vi "Shock&Dyanamics Laboratory - DROPBEAR_June2022_Rev3.vi"() -> ()   [LabVIEW 2019] (continued)
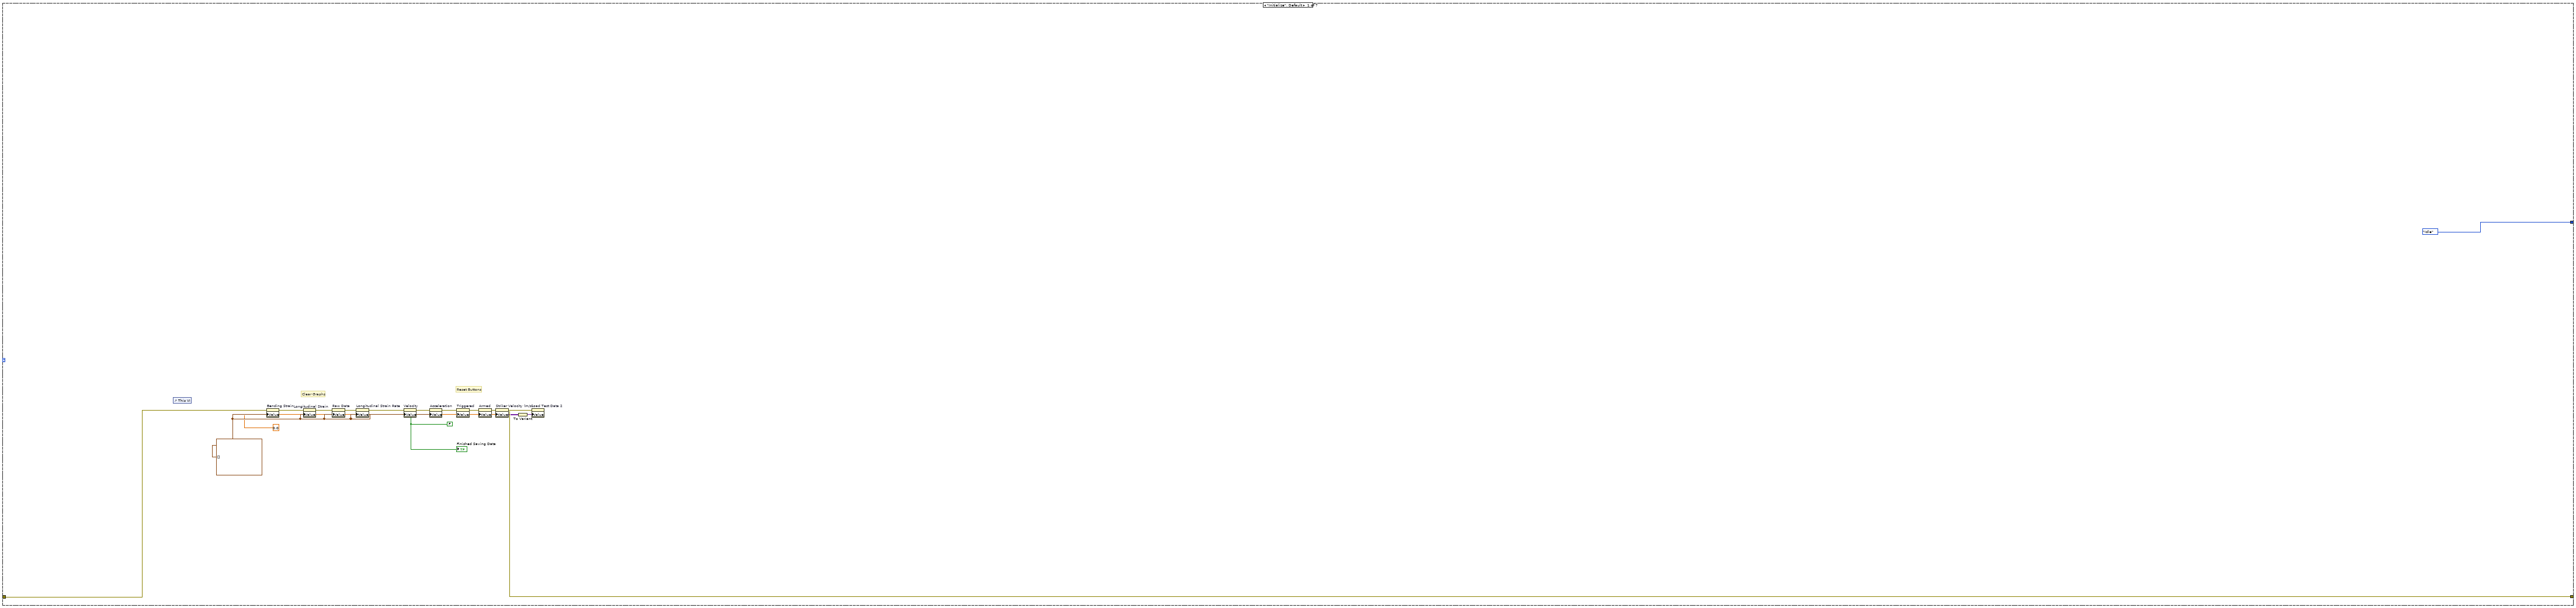
[diagram p2: hidden frame]
                # "== Need to change save file to accuratly save the sperated and strain-rate Data =="
                n2032 = Two Button Dialog(message="Use the folder/file names already given?", 1:"No" ("F button name (\"Cancel\")"), 2:"Yes" ("T button name (\"OK\")")) -> (T button?=w2561:bool)
                n2033 = case shown="True" w2561 {
                  tunnel: [w2582 "Folder Name to Save Raw Data"] -> w2560
                  tunnel: [w2581 "File Name to Save Raw Data"] -> w2559
                  tunnel: w2558 -> [w2579 w2583]
                  tunnel: [w2578 w2583] -> w2557
                  frame False {
                    n2034 = call "32CHDAQ - New FileFolder Names.vi"("Enable"=TRUE, "error in (no error)"=w2579) -> ("File Name (don't forget .txt)"=w2581:string, "Folder Name"=w2582:string, "error out"=w2578:errorcluster)  [unwired: 14 in, 1 out]
                  }
                  frame True {
                  }
                }
                n2035 = flat-sequence {
                  tunnel: w2557 -> [w2586]
                  tunnel: w2559 -> [w2587]
                  tunnel: w2560 -> [w2588]
                  tunnel: [w2588] -> w2572
                  tunnel: [w2587] -> w2571
                  tunnel: [w2586] -> w2570
                  tunnel: [w2592] -> w2556
                  tunnel: [w2594] -> w2554
                  tunnel: [w2593] -> w2552
                  tunnel: w2572 -> [w2594]
                  tunnel: w2571 -> [w2593]
                  tunnel: w2570 -> [w2591]
                  tunnel: w2573 -> [w2590]
                  tunnel: [w2590] -> w2550
                  tunnel: w2556 -> [w2609]
                  tunnel: [w2608] -> w2555
                  tunnel: w2554 -> [w2606]
                  tunnel: [w2606] -> w2553
                  tunnel: w2552 -> [w2607]
                  tunnel: [w2607] -> w2551
                  tunnel: w2550 -> [w2605]
                  tunnel: [w2605] -> w2549
                  tunnel: "Incident Name for First Pulse\n(Must Match Exactly" -> [w2604]
                  tunnel: w2555 -> [w2628]
                  tunnel: w2553 -> [w2623]
                  tunnel: w2551 -> [w2629]
                  tunnel: [w2623] -> w2569
                  tunnel: [w2629] -> w2568
                  tunnel: [w2627] -> w2567
                  tunnel: w2549 -> [w2626]
                  tunnel: [w2626] -> w2566
                  tunnel: "Incident Name for First Pulse\n(Must Match Exactly" -> [w2624]
                  tunnel: w2569 -> [w2659]
                  tunnel: w2568 -> [w2658]
                  tunnel: [w2659] -> w2565
                  tunnel: [w2658] -> w2564
                  tunnel: [w2656] -> w2563
                  tunnel: w2567 -> [w2657]
                  tunnel: w2566 -> [w2655]
                  tunnel: [w2655] -> w2562
                  tunnel: w2565 -> [w2678]
                  tunnel: w2564 -> [w2677]
                  tunnel: w2563 -> [w2676]
                  tunnel: [w2675] -> w2574
                  tunnel: w2562 -> [w2674]
                  frame #0 {
                  }
                  frame #1 {
                    w2589 = TRUE
                    # "Saves Raw Data"
                    n2036 = case shown="True" w2589 {
                      tunnel: w2594 -> [_ w2603]
                      tunnel: w2593 -> [_ w2602]
                      tunnel: [w2595 w2601] -> w2592
                      tunnel: w2591 -> [w2595 w2599]
                      tunnel: w2590 -> [_ w2597]
                      frame False {
                      }
                      frame True {
                        n2037 = property on="Raw Data" class="WFGraph (strict)"() -> ("Value"=w2596:waveform(dbl)[])  [unwired: 2 in, 2 out]
                        n2038 = property on="Save Info" class="Clust (strict)"() -> ("Value"=w2598:T5)  [unwired: 2 in, 2 out]
                        n2039 = Concatenate Strings(w2603, w2602) -> (w2600:string)
                        n2040 = call "32CHDAQ - Save Data File 0 Raw.vi"("Save Info"=w2598, "error in"=w2599, "waveforms"=w2596, "output cluster 3"=w2597, "File name"=w2600) -> ("error out"=w2601:errorcluster)  [unwired: 6 in]
                      }
                    }
                    "?" <- w2589
                  }
                  frame #2 {
                    # "Saves First Pulse of Raw Data"
                    n2041 = case shown="True" "First Pulse" {
                      tunnel: w2609 -> [w2611 w2621]
                      tunnel: [w2611 w2620] -> w2608
                      tunnel: w2607 -> [_ w2617]
                      tunnel: w2606 -> [_ w2616]
                      tunnel: w2605 -> [_ w2615]
                      tunnel: w2604 -> [_ w2612]
                      frame False {
                      }
                      frame True {
                        # "Save First Pulse Only subVI"
                        n2042 = property on="Raw Data" class="WFGraph (strict)"() -> ("Value"=w2613:waveform(dbl)[])  [unwired: 2 in, 2 out]
                        n2043 = Concatenate Strings(w2616, "First_Pulse_" ("string"), w2617) -> (w2618:string)
                        n2044 = property on="Save Info" class="Clust (strict)"() -> ("Value"=w2614:T5)  [unwired: 2 in, 2 out]
                        n2045 = call "32CHDAQ - Save Data File - FirstPulse.vi"("Incident Name for First Pulse\n(Must Match Exactly"=w2612, "Save Info"=w2614, "error in"=w2621, "waveforms"=w2613, "output cluster 3"=w2615, "File name"=w2618) -> ("error out"=w2620:errorcluster)  [unwired: 5 in]
                      }
                    }
                  }
                  frame #3 {
                    n2046 = property on="First Pulse" class="Bool (strict)"() -> ("Value"=w2622:bool)  [unwired: 2 in, 2 out]
                    n2047 = case shown="True" "?" {
                      tunnel: w2623 -> [_ w2635]
                      tunnel: w2629 -> [_ w2636]
                      tunnel: w2628 -> [w2630 w2640]
                      tunnel: [w2630 w2639] -> w2627
                      tunnel: w2626 -> [_ w2632]
                      tunnel: w2624 -> [_ w2637]
                      tunnel: w2622 -> [_ w2631]
                      frame False {
                      }
                      frame True {
                        (unwired) "Scaled Data" ("Comment")
                        n2048 = property on="Scaled Data" class="Arr (strict)"() -> ("Value"=w2634:waveform(dbl)[])  [unwired: 2 in, 2 out]
                        n2049 = Concatenate Strings(w2635, "True_" ("string"), w2636) -> (w2641:string)
                        n2050 = property on="Save Info" class="Clust (strict)"() -> ("Value"=w2633:T5)  [unwired: 2 in, 2 out]
                        n2051 = call "32CHDAQ - Save Data File.vi"("Save Info"=w2633, "error in"=w2640, "waveforms"=w2634, "output cluster 3"=w2632, "File name"=w2641) -> ("error out"=w2638:errorcluster)  [unwired: 6 in]
                        n2052 = case shown="True" w2631 {
                          tunnel: w2638 -> [w2643 w2653]
                          tunnel: [w2643 w2652] -> w2639
                          tunnel: w2636 -> [_ w2649]
                          tunnel: w2635 -> [_ w2648]
                          tunnel: w2632 -> [_ w2647]
                          tunnel: w2637 -> [_ w2646]
                          tunnel: w2634 -> [_ w2645]
                          tunnel: w2633 -> [_ w2644]
                          frame False {
                          }
                          frame True {
                            # "Save First Pulse Only subVI"
                            n2053 = Concatenate Strings(w2648, "First_Pulse_Scaled_" ("string"), w2649) -> (w2650:string)
                            n2054 = call "32CHDAQ - Save Data File - FirstPulse.vi"("Incident Name for First Pulse\n(Must Match Exactly"=w2646, "Save Info"=w2644, "error in"=w2653, "waveforms"=w2645, "output cluster 3"=w2647, "File name"=w2650) -> ("error out"=w2652:errorcluster)  [unwired: 5 in]
                          }
                        }
                      }
                    }
                  }
                  frame #4 {
                    # "Saves Separated Data - Turned Off Right Now"
                    n2055 = case shown="True" "Separated" {
                      tunnel: w2659 -> [_ w2671]
                      tunnel: w2658 -> [_ w2670]
                      tunnel: w2657 -> [w2660 w2666]
                      tunnel: [w2660 w2665] -> w2656
                      tunnel: w2655 -> [_ w2661]
                      frame False {
                      }
                      frame True {
                        (unwired) "Seperated Data" ("Comment")
                        n2056 = property on="Bending Strain" class="WFGraph (strict)"() -> ("Value"=w2668:waveform(dbl)[])  [unwired: 2 in, 2 out]
                        n2057 = Concatenate Strings(w2671, "Sep_" ("string"), w2670) -> (w2663:string)
                        n2058 = property on="Longitudinal Strain" class="WFGraph (strict)"() -> ("Value"=w2669:waveform(dbl)[])  [unwired: 2 in, 2 out]
                        n2059 = Insert Into Array(array=waveform(dbl)[] [], new element #1=w2668, new element #2=w2669) -> (w2664:waveform(dbl)[])  [unwired: 1 in]
                        n2060 = property on="Save Info" class="Clust (strict)"() -> ("Value"=w2662:T5)  [unwired: 2 in, 2 out]
                        n2061 = call "32CHDAQ - Save Data File - Seperated.vi"("Save Info"=w2662, "error in"=w2666, "waveforms"=w2664, "output cluster 3"=w2661, "File name"=w2663) -> ("error out"=w2665:errorcluster)  [unwired: 6 in]
                      }
                    }
                  }
                  frame #5 {
                    # "Save Strain-Rate Data - Turned Off Right Now"
                    n2062 = case shown="True" "?" {
                      tunnel: w2678 -> [_ w2688]
                      tunnel: w2677 -> [_ w2687]
                      tunnel: w2676 -> [w2679 w2684]
                      tunnel: [w2679 w2683] -> w2675
                      tunnel: w2674 -> [_ w2681]
                      frame False {
                      }
                      frame True {
                        (unwired) "Strain Rate Data" ("Comment")
                        n2063 = Concatenate Strings(w2688, "Rate_" ("string"), w2687) -> (w2686:string)
                        n2064 = property on="Rate Data" class="Arr (strict)"() -> ("Value"=w2680:waveform(dbl)[])  [unwired: 2 in, 2 out]
                        n2065 = property on="Save Info" class="Clust (strict)"() -> ("Value"=w2685:T5)  [unwired: 2 in, 2 out]
                        n2066 = case shown="False" FALSE {
                          tunnel: w2686 -> [_ w2696]
                          tunnel: w2685 -> [_ w2695]
                          tunnel: w2680 -> [_ w2691]
                          tunnel: w2684 -> [w2690 w2694]
                          tunnel: [w2690 w2693] -> w2683
                          tunnel: w2681 -> [_ w2692]
                          frame False {
                          }
                          frame True {
                            n2067 = call "32CHDAQ - Save Data File - Rate.vi"("Save Info"=w2695, "error in"=w2694, "waveforms"=w2691, "output cluster 3"=w2692, "File name"=w2696) -> ("error out"=w2693:errorcluster)  [unwired: 6 in]
                          }
                        }
                      }
                    }
                  }
                }
              }
            }
            n2068 = property on="Finished Saving Data" class="Bool (strict)"(error in=w2543, "Value"=TRUE ("Finished Saving Data")) -> (error out=w2541:errorcluster)  [unwired: 1 in, 1 out]
            n2069 = property on="Triggered" class="Bool (strict)"(error in=w2541, "Value"=FALSE ("Triggered")) -> (error out=w2539:errorcluster)  [unwired: 1 in, 1 out]
            n2070 = flat-sequence {
              tunnel: w2539 -> [w2697]
              tunnel: [w2697] -> w2538
              frame #0 {
                n2071 = Wait (ms)(milliseconds to wait=u32 1000) -> ()  [unwired: 1 out]
              }
            }
          }
          frame "Load Data" {
            n2072 = Two Button Dialog(message="Have you loaded the associated Channel Data file?\n(if not, do so before loading the Test Data File)     ", 1:"No" ("F button name (\"Cancel\")"), 2:"Yes" ("T button name (\"OK\")")) -> (T button?=w2703:bool)
            n2073 = case shown="True" w2703 {
              tunnel: [32CHDAQ_-_Cases."Idle" ("Program State") 32CHDAQ_-_Cases."Process Data" ("Program State")] -> w2702
              frame False {
                n2074 = To Variant(anything=FALSE) -> (Variant=w2707:variant)
                n2075 = property on="Load Test Data 2" class="Bool"("Value"=w2707) -> ()  [unwired: 2 in, 2 out]
              }
              frame True {
                w2723 = T58 1 items=["no dialog", "OK message", "continue or stop message", "OK message + warnings", "continue/stop + warnings"] ("type of dialog (OK msg:1)")
                # "Prompt User to Load Test Data File"
                n2076 = property on="output cluster" class="Clust (strict)"() -> (error out=w2714:errorcluster, "Value"=w2715:T2)  [unwired: 2 in, 1 out]
                n2077 = property on="Folder Name to Save Raw Data" class="Str"() -> ("Value"=w2732:string)  [unwired: 2 in, 2 out]
                n2078 = Unbundle(w2715) -> (w2720:T59, w2719:T60)  [unwired: 10 out]
                n2079 = Cluster To Array(cluster=w2720) -> (array=w2716:bool[])
                n2080 = Cluster To Array(cluster=w2719) -> (array=w2718:string[])
                n2081 = String To Path(string=w2732) -> (path=w2733:path)
                n2082 = File Dialog(4:"TXT File" ("pattern label"), 6:"*.txt" ("pattern"), 7:"Load Channel Data File" ("prompt"), 9:"*.txt" ("default name"), 11:w2733) -> (3:w2709:path)  [unwired: 2 in, 3 out]
                n2083 = call-poly <vilib>:"Read Delimited Spreadsheet.vi"("file path (dialog if empty)"=w2709) -> ("all rows"=w2708:dbl[][])  [unwired: 9 in, 5 out]
                n2084 = Transpose 2D Array(2D array=w2708) -> (transposed array=w2712:dbl[][])
                n2085 = Delete From Array(array=w2712, length=9, index (col)=0 ("index")) -> (array with subset deleted=w2711:dbl[][])  [unwired: 1 in, 1 out]
                n2086 = for {
                  tunnel: w2718 -> [w2741] mode=indexing
                  shift-right: [w2740] -> w2727
                  shift-left: string[] [] -> [w2739]
                  tunnel: w2716 -> [w2738] mode=indexing
                  n2087 = case shown="True" w2738 {
                    tunnel: w2741 -> [_ w2743]
                    tunnel: [w2742 w2745] -> w2740
                    tunnel: w2739 -> [w2742 w2744]
                    frame False {
                    }
                    frame True {
                      n2088 = Build Array (concatenate)(w2744, w2743) -> (w2745:string[])
                    }
                  }
                }
                n2089 = property on="Sample Rate (Sa/sec)" class="DigNum (strict)"(error in=w2714) -> (error out=w2726:errorcluster, "Value"=w2731:dbl)  [unwired: 1 in, 1 out]
                n2090 = for {
                  N -> [w2752]
                  tunnel: w2711 -> [w2755] mode=indexing
                  tunnel: w2731 -> [w2753]
                  tunnel: [w2750] -> w2730 mode=indexing
                  tunnel: [w2752] -> w2729
                  tunnel: w2727 -> [w2748] mode=indexing
                  shift-right: [w2746] -> w2725
                  shift-left: w2726 -> [w2747]
                  n2091 = Reciprocal(x=w2753) -> (1/x=w2754:dbl)
                  n2092 = Bundle By Name("dt"=w2754, "Y"=w2755) -> (w2751:waveform(dbl))  [unwired: 1 in]
                  n2093 = Set Waveform Attribute(4:w2747, 5:w2748, 6:"NI_ChannelName" ("name"), 7:w2751) -> (0:w2746:errorcluster, 3:w2750:waveform(dbl))  [unwired: 1 out]
                }
                n2094 = property on="Raw Data" class="WFGraph (strict)"(error in=w2725, "Value"=w2730) -> (error out=w2724:errorcluster)  [unwired: 1 in, 1 out]
                n2095 = Decrement(x=w2729) -> (x-1=w2728:i32)
                n2096 = property on="Number of Channels" class="DigNum (strict)"(error in=w2724, "Value"=w2728) -> (error out=w2722:errorcluster)  [unwired: 1 in, 1 out]
                n2097 = call <vilib>:"Simple Error Handler.vi"("type of dialog (OK msg:1)"=w2723, "error in (no error)"=w2722) -> ()  [unwired: 3 in, 5 out]
              }
            }
          }
          frame "End" {
            w2757 = FALSE ("Finished Saving Data")
            w2759 = waveform(dbl)[] [] ("array")
            # "Reset Buttons"
            # "Clear  Graphs"
            # "This is just a placeholder"
            # "Tie Up any Loose ends before ending Program"
            n2098 = property on="Raw Data" class="WFGraph (strict)"(error in=w2766, "Value"=w2759) -> (error out=w2765:errorcluster)  [unwired: 1 in, 1 out]
            n2099 = property on="Longitudinal Strain" class="WFGraph (strict)"(error in=w2765, "Value"=w2759) -> (error out=w2764:errorcluster)  [unwired: 1 in, 1 out]
            n2100 = property on="Bending Strain" class="WFGraph (strict)"(error in=w2764, "Value"=w2759) -> (error out=w2763:errorcluster)  [unwired: 1 in, 1 out]
            n2101 = property on="Longitudinal Strain Rate" class="WFGraph (strict)"(error in=w2763, "Value"=w2759) -> (error out=w2762:errorcluster)  [unwired: 1 in, 1 out]
            n2102 = property on="Velocity" class="WFGraph (strict)"(error in=w2762, "Value"=w2759) -> (error out=w2761:errorcluster)  [unwired: 1 in, 1 out]
            n2103 = property on="Acceleration" class="WFGraph (strict)"(error in=w2761, "Value"=w2759) -> (error out=w2760:errorcluster)  [unwired: 1 in, 1 out]
            n2104 = property on="Finished Saving Data" class="Bool (strict)"(error in=w2760, "Value"=w2757) -> (error out=w2767:errorcluster)  [unwired: 1 in, 1 out]
            n2105 = call <vilib>:"Simple Error Handler.vi"("error in (no error)"=w2767) -> ("error out"=w2758:errorcluster)  [unwired: 4 in, 4 out]
            "Triggered" <- w2757
            "Armed" <- w2757
          }
        }
      }
      frame #1 {
        # "Add \nProperty\nNode\nHere"
        # "Gather Channel Information"
        n2106 = Bundle("Sens Fac 0"="Sens Fac 0", "Sens Fac 1"="Sens Fac 1", "Sens Fac 2"="Sens Fac 2", "Sens Fac 3"="Sens Fac 3", "Sens Fac 4"="Sens Fac 4", "Sens Fac 5"="Sens Fac 5", "Sens Fac 6"="Sens Fac 6", "Sens Fac 7"="Sens Fac 7", "Sens Fac 8"="Sens Fac 8", "Sens Fac 9"="Sens Fac 9", "Sens Fac 10"="Sens Fac 10", "Sens Fac 11"="Sens Fac 11", "Sens Fac 12"="Sens Fac 12", "Sens Fac 13"="Sens Fac 13", "Sens Fac 14"="Sens Fac 14", "Sens Fac 15"="Sens Fac 15", "Sens Fac 16"="Sens Fac 16", "Sens Fac 17"="Sens Fac 17", "Sens Fac 18"="Sens Fac 18", "Sens Fac 19"="Sens Fac 19", "Sens Fac 20"="Sens Fac 20", "Sens Fac 21"="Sens Fac 21", "Sens Fac 22"="Sens Fac 22", "Sens Fac 23"="Sens Fac 23", "Sens Fac 24"="Sens Fac 24", "Sens Fac 25"="Sens Fac 25", "Sens Fac 26"="Sens Fac 26", "Sens Fac 27"="Sens Fac 27", "Sens Fac 28"="Sens Fac 28", "Sens Fac 29"="Sens Fac 29", "Sens Fac 30"="Sens Fac 30", "Sens Fac 31"="Sens Fac 31") -> (w2984:T51)  [unwired: 1 in]
        n2107 = Bundle(TRUE, "Enable Ch 1"="Enable Ch 1", "Enable Ch 2"="Enable Ch 2", "Enable Ch 3"="Enable Ch 3", "Enable Ch 4"="Enable Ch 4", "Enable Ch 5"="Enable Ch 5", "Enable Ch 6"="Enable Ch 6", "Enable Ch 7"="Enable Ch 7", "Enable Ch 8"="Enable Ch 8", "Enable Ch 9"="Enable Ch 9", "Enable Ch 10"="Enable Ch 10", "Enable Ch 11"="Enable Ch 11", "Enable Ch 12"="Enable Ch 12", "Enable Ch 13"="Enable Ch 13", "Enable Ch 14"="Enable Ch 14", "Enable Ch 15"="Enable Ch 15", "Enable Ch 16"="Enable Ch 16", "Enable Ch 17"="Enable Ch 17", "Enable Ch 18"="Enable Ch 18", "Enable Ch 19"="Enable Ch 19", "Enable Ch 20"="Enable Ch 20", "Enable Ch 21"="Enable Ch 21", "Enable Ch 22"="Enable Ch 22", "Enable Ch 23"="Enable Ch 23", "Enable Ch 24"="Enable Ch 24", "Enable Ch 25"="Enable Ch 25", "Enable Ch 26"="Enable Ch 26", "Enable Ch 27"="Enable Ch 27", "Enable Ch 28"="Enable Ch 28", "Enable Ch 29"="Enable Ch 29", "Enable Ch 30"="Enable Ch 30", "Enable Ch 31"="Enable Ch 31") -> (w2989:T59)  [unwired: 1 in]
        "ON/OFF" <- w2989
        n2108 = Bundle("SG Pair Ch 0"="SG Pair Ch 0", "SG Pair Ch 1"="SG Pair Ch 1", "SG Pair Ch 2"="SG Pair Ch 2", "SG Pair Ch 3"="SG Pair Ch 3", "SG Pair Ch 4"="SG Pair Ch 4", "SG Pair Ch 5"="SG Pair Ch 5", "SG Pair Ch 6"="SG Pair Ch 6", "SG Pair Ch 7"="SG Pair Ch 7", "SG Pair Ch 8"="SG Pair Ch 8", "SG Pair Ch 9"="SG Pair Ch 9", "SG Pair Ch 10"="SG Pair Ch 10", "SG Pair Ch 11"="SG Pair Ch 11", "SG Pair Ch 12"="SG Pair Ch 12", "SG Pair Ch 13"="SG Pair Ch 13", "SG Pair Ch 14"="SG Pair Ch 14", "SG Pair Ch 15"="SG Pair Ch 15", "SG Pair Ch 16"="SG Pair Ch 16", "SG Pair Ch 17"="SG Pair Ch 17", "SG Pair Ch 18"="SG Pair Ch 18", "SG Pair Ch 19"="SG Pair Ch 19", "SG Pair Ch 20"="SG Pair Ch 20", "SG Pair Ch 21"="SG Pair Ch 21", "SG Pair Ch 22"="SG Pair Ch 22", "SG Pair Ch 23"="SG Pair Ch 23", "SG Pair Ch 24"="SG Pair Ch 24", "SG Pair Ch 25"="SG Pair Ch 25", "SG Pair Ch 26"="SG Pair Ch 26", "SG Pair Ch 27"="SG Pair Ch 27", "SG Pair Ch 28"="SG Pair Ch 28", "SG Pair Ch 29"="SG Pair Ch 29", "SG Pair Ch 30"="SG Pair Ch 30", "SG Pair Ch 31"="SG Pair Ch 31") -> (w2981:T53)  [unwired: 1 in]
        n2109 = Bundle("Voltage Max Ch 0"="Voltage Max Ch 0", "Voltage Max Ch 1"="Voltage Max Ch 1", "Voltage Max Ch 2"="Voltage Max Ch 2", "Voltage Max Ch 3"="Voltage Max Ch 3", "Voltage Max Ch 4"="Voltage Max Ch 4", "Voltage Max Ch 5"="Voltage Max Ch 5", "Voltage Max  Ch 6"="Voltage Max  Ch 6", "Voltage Max Ch 7"="Voltage Max Ch 7", "Voltage Max Ch 8"="Voltage Max Ch 8", "Voltage Max Ch 9"="Voltage Max Ch 9", "Voltage Max Ch 10"="Voltage Max Ch 10", "Voltage Max Ch 11"="Voltage Max Ch 11", "Voltage Max Ch 12"="Voltage Max Ch 12", "Voltage Max Ch 13"="Voltage Max Ch 13", "Voltage Max Ch 14"="Voltage Max Ch 14", "Voltage Max Ch 15"="Voltage Max Ch 15", "Voltage Max Ch 16"="Voltage Max Ch 16", "Voltage Max Ch 17"="Voltage Max Ch 17", "Voltage Max Ch 18"="Voltage Max Ch 18", "Voltage Max Ch 19"="Voltage Max Ch 19", "Voltage Max Ch 20"="Voltage Max Ch 20", "Voltage Max Ch 21"="Voltage Max Ch 21", "Voltage Max Ch 22"="Voltage Max Ch 22", "Voltage Max Ch 23"="Voltage Max Ch 23", "Voltage Max Ch 24"="Voltage Max Ch 24", "Voltage Max Ch 25"="Voltage Max Ch 25", "Voltage Max Ch 26"="Voltage Max Ch 26", "Voltage Max Ch 27"="Voltage Max Ch 27", "Voltage Max Ch 28"="Voltage Max Ch 28", "Voltage Max Ch 29"="Voltage Max Ch 29", "Voltage Max Ch 30"="Voltage Max Ch 30", "Voltage Max Ch 31"="Voltage Max Ch 31") -> (w2986:T61)  [unwired: 1 in]
        n2110 = Bundle("SG Pair 0"="SG Pair 0", "SG Pair 1"="SG Pair 1", "SG Pair 2"="SG Pair 2", "SG Pair 3"="SG Pair 3", "SG Pair 4"="SG Pair 4", "SG Pair 5"="SG Pair 5", "SG Pair 6"="SG Pair 6", "SG Pair 7"="SG Pair 7", "SG Pair 8"="SG Pair 8", "SG Pair 9"="SG Pair 9", "SG Pair 10"="SG Pair 10", "SG Pair 11"="SG Pair 11", "SG Pair 12"="SG Pair 12", "SG Pair 13"="SG Pair 13", "SG Pair 14"="SG Pair 14", "SG Pair 15"="SG Pair 15", "SG Pair 16"="SG Pair 16", "SG Pair 17"="SG Pair 17", "SG Pair 18"="SG Pair 18", "SG Pair 19"="SG Pair 19", "SG Pair 20"="SG Pair 20", "SG Pair 21"="SG Pair 21", "SG Pair 22"="SG Pair 22", "SG Pair 23"="SG Pair 23", "SG Pair 24"="SG Pair 24", "SG Pair 25"="SG Pair 25", "SG Pair 26"="SG Pair 26", "SG Pair 27"="SG Pair 27", "SG Pair 28"="SG Pair 28", "SG Pair 29"="SG Pair 29", "SG Pair 30"="SG Pair 30", "SG Pair 31"="SG Pair 31") -> (w2982:T52)  [unwired: 1 in]
        n2111 = Bundle("Name (Laser Gate)"="Name (Laser Gate)", "Name Ch 1"="Name Ch 1", "Name Ch 2"="Name Ch 2", "Name Ch 3"="Name Ch 3", "Name Ch 4"="Name Ch 4", "Name Ch 5"="Name Ch 5", "Name Ch 6"="Name Ch 6", "Name Ch 7"="Name Ch 7", "Name Ch 8"="Name Ch 8", "Name Ch 9"="Name Ch 9", "Name Ch 10"="Name Ch 10", "Name Ch 11"="Name Ch 11", "Name Ch 12"="Name Ch 12", "Name Ch 13"="Name Ch 13", "Name Ch 14"="Name Ch 14", "Name Ch 15"="Name Ch 15", "Name Ch 16"="Name Ch 16", "Name Ch 17"="Name Ch 17", "Name Ch 18"="Name Ch 18", "Name Ch 19"="Name Ch 19", "Name Ch 20"="Name Ch 20", "Name Ch 21"="Name Ch 21", "Name Ch 22"="Name Ch 22", "Name Ch 23"="Name Ch 23", "Name Ch 24"="Name Ch 24", "Name Ch 25"="Name Ch 25", "Name Ch 26"="Name Ch 26", "Name Ch 27"="Name Ch 27", "Name Ch 28"="Name Ch 28", "Name Ch 29"="Name Ch 29", "Name Ch 30"="Name Ch 30", "Name Ch 31"="Name Ch 31") -> (w2990:T60)  [unwired: 1 in]
        n2112 = Bundle("Voltage Min Ch 0"="Voltage Min Ch 0", "Voltage Min Ch 1"="Voltage Min Ch 1", "Voltage Min Ch 2"="Voltage Min Ch 2", "Voltage Min Ch 3"="Voltage Min Ch 3", "Voltage Min Ch 4"="Voltage Min Ch 4", "Voltage Min Ch 5"="Voltage Min Ch 5", "Voltage Min Ch 6"="Voltage Min Ch 6", "Voltage Min Ch 7"="Voltage Min Ch 7", "Voltage Min Ch 8"="Voltage Min Ch 8", "Voltage Min Ch 9"="Voltage Min Ch 9", "Voltage Min Ch 10"="Voltage Min Ch 10", "Voltage Min Ch 11"="Voltage Min Ch 11", "Voltage Min Ch 12"="Voltage Min Ch 12", "Voltage Min Ch 13"="Voltage Min Ch 13", "Voltage Min Ch 14"="Voltage Min Ch 14", "Voltage Min Ch 15"="Voltage Min Ch 15", "Voltage Min Ch 16"="Voltage Min Ch 16", "Voltage Min Ch 17"="Voltage Min Ch 17", "Voltage Min Ch 18"="Voltage Min Ch 18", "Voltage Min Ch 19"="Voltage Min Ch 19", "Voltage Min Ch 20"="Voltage Min Ch 20", "Voltage Min Ch 21"="Voltage Min Ch 21", "Voltage Min Ch 22"="Voltage Min Ch 22", "Voltage Min Ch 23"="Voltage Min Ch 23", "Voltage Min Ch 24"="Voltage Min Ch 24", "Voltage Min Ch 25"="Voltage Min Ch 25", "Voltage Min Ch 26"="Voltage Min Ch 26", "Voltage Min Ch 27"="Voltage Min Ch 27", "Voltage Min Ch 28"="Voltage Min Ch 28", "Voltage Min Ch 29"="Voltage Min Ch 29", "Voltage Min Ch 30"="Voltage Min Ch 30", "Voltage Min Ch 31"="Voltage Min Ch 31") -> (w2987:T62)  [unwired: 1 in]
        n2113 = Bundle("Signal Type 0"="Signal Type 0", "Signal Type 1"="Signal Type 1", "Signal Type 2"="Signal Type 2", "Signal Type 3"="Signal Type 3", "Signal Type 4"="Signal Type 4", "Signal Type 5"="Signal Type 5", "Signal Type 6"="Signal Type 6", "Signal Type 7"="Signal Type 7", "Signal Type 8"="Signal Type 8", "Signal Type 9"="Signal Type 9", "Signal Type 10"="Signal Type 10", "Signal Type 11"="Signal Type 11", "Signal Type 12"="Signal Type 12", "Signal Type 13"="Signal Type 13", "Signal Type 14"="Signal Type 14", "Signal Type 15"="Signal Type 15", "Signal Type 16"="Signal Type 16", "Signal Type 17"="Signal Type 17", "Signal Type 18"="Signal Type 18", "Signal Type 19"="Signal Type 19", "Signal Type 20"="Signal Type 20", "Signal Type 21"="Signal Type 21", "Signal Type 22"="Signal Type 22", "Signal Type 23"="Signal Type 23", "Signal Type 24"="Signal Type 24", "Signal Type 25"="Signal Type 25", "Signal Type 26"="Signal Type 26", "Signal Type 27"="Signal Type 27", "Signal Type 28"="Signal Type 28", "Signal Type 29"="Signal Type 29", "Signal Type 30"="Signal Type 30", "Signal Type 31"="Signal Type 31") -> (w2983:T4)  [unwired: 1 in]
        "Signal Type" <- w2983
        n2114 = call "16CHDAQ - PF Info Num2Str.vi"("PF Channel"="PF Card 0", "PF Card"="PF Channel 0", "PF Chassis"="PF Chassis 0") -> ("PF Info"=w3152:string)
        n2115 = call "16CHDAQ - PF Info Num2Str.vi"("PF Channel"="PF Card 1", "PF Card"="PF Channel 1", "PF Chassis"="PF Chassis 1") -> ("PF Info"=w3156:string)
        n2116 = call "16CHDAQ - PF Info Num2Str.vi"("PF Channel"="PF Channel 2", "PF Card"="PF Card 2", "PF Chassis"="PF Chassis 2") -> ("PF Info"=w3162:string)
        n2117 = call "16CHDAQ - PF Info Num2Str.vi"("PF Channel"="PF Channel 3", "PF Card"="PF Card 3", "PF Chassis"="PF Chassis 3") -> ("PF Info"=w3166:string)
        n2118 = call "16CHDAQ - PF Info Num2Str.vi"("PF Channel"="PF Channel 4", "PF Card"="PF Card 4", "PF Chassis"="PF Chassis 4") -> ("PF Info"=w3170:string)
        n2119 = call "16CHDAQ - PF Info Num2Str.vi"("PF Channel"="PF Channel 5", "PF Card"="PF Card 5", "PF Chassis"="PF Chassis 5") -> ("PF Info"=w3174:string)
        n2120 = call "16CHDAQ - PF Info Num2Str.vi"("PF Channel"="PF Channel 6", "PF Card"="PF Card 6", "PF Chassis"="PF Chassis 6") -> ("PF Info"=w3178:string)
        n2121 = call "16CHDAQ - PF Info Num2Str.vi"("PF Channel"="PF Channel 7", "PF Card"="PF Card 7", "PF Chassis"="PF Chassis 7") -> ("PF Info"=w3182:string)
        n2122 = call "16CHDAQ - PF Info Num2Str.vi"("PF Channel"="PF Channel 8", "PF Card"="PF Card 8", "PF Chassis"="PF Chassis 8") -> ("PF Info"=w3186:string)
        n2123 = call "16CHDAQ - PF Info Num2Str.vi"("PF Channel"="PF Channel 9", "PF Card"="PF Card 9", "PF Chassis"="PF Chassis 9") -> ("PF Info"=w3215:string)
        n2124 = call "16CHDAQ - PF Info Num2Str.vi"("PF Channel"="PF Channel 10", "PF Card"="PF Card 10", "PF Chassis"="PF Chassis 10") -> ("PF Info"=w3216:string)
        n2125 = call "16CHDAQ - PF Info Num2Str.vi"("PF Channel"="PF Channel 11", "PF Card"="PF Card 11", "PF Chassis"="PF Chassis 11") -> ("PF Info"=w3217:string)
        n2126 = call "16CHDAQ - PF Info Num2Str.vi"("PF Channel"="PF Channel 12", "PF Card"="PF Card 12", "PF Chassis"="PF Chassis 12") -> ("PF Info"=w3218:string)
        n2127 = call "16CHDAQ - PF Info Num2Str.vi"("PF Channel"="PF Channel 13", "PF Card"="PF Card 13", "PF Chassis"="PF Chassis 13") -> ("PF Info"=w3219:string)
        n2128 = call "16CHDAQ - PF Info Num2Str.vi"("PF Channel"="PF Channel 14", "PF Card"="PF Card 14", "PF Chassis"="PF Chassis 14") -> ("PF Info"=w3220:string)
        n2129 = call "16CHDAQ - PF Info Num2Str.vi"("PF Channel"="PF Channel 15", "PF Card"="PF Card 15", "PF Chassis"="PF Chassis 15") -> ("PF Info"=w3221:string)
        n2130 = call "16CHDAQ - PF Info Num2Str.vi"("PF Channel"="PF Channel 16", "PF Card"="PF Card 16", "PF Chassis"="PF Chassis 16") -> ("PF Info"=w2819:string)
        n2131 = call "16CHDAQ - PF Info Num2Str.vi"("PF Channel"="PF Channel 17", "PF Card"="PF Card 17", "PF Chassis"="PF Chassis 17") -> ("PF Info"=w2818:string)
        n2132 = call "16CHDAQ - PF Info Num2Str.vi"("PF Channel"="PF Channel 18", "PF Card"="PF Card 18", "PF Chassis"="PF Chassis 18") -> ("PF Info"=w2817:string)
        n2133 = call "16CHDAQ - PF Info Num2Str.vi"("PF Channel"="PF Channel 19", "PF Card"="PF Card 19", "PF Chassis"="PF Chassis 19") -> ("PF Info"=w2816:string)
        n2134 = call "16CHDAQ - PF Info Num2Str.vi"("PF Channel"="PF Channel 20", "PF Card"="PF Card 20", "PF Chassis"="PF Chassis 20") -> ("PF Info"=w2815:string)
        n2135 = call "16CHDAQ - PF Info Num2Str.vi"("PF Channel"="PF Channel 21", "PF Card"="PF Card 21", "PF Chassis"="PF Chassis 21") -> ("PF Info"=w2814:string)
        n2136 = call "16CHDAQ - PF Info Num2Str.vi"("PF Channel"="PF Channel 22", "PF Card"="PF Card 22", "PF Chassis"="PF Chassis 22") -> ("PF Info"=w2813:string)
        n2137 = call "16CHDAQ - PF Info Num2Str.vi"("PF Channel"="PF Channel 23", "PF Card"="PF Card 23", "PF Chassis"="PF Chassis 23") -> ("PF Info"=w2812:string)
        n2138 = call "16CHDAQ - PF Info Num2Str.vi"("PF Channel"="PF Channel 24", "PF Card"="PF Card 24", "PF Chassis"="PF Chassis 24") -> ("PF Info"=w2811:string)
        n2139 = call "16CHDAQ - PF Info Num2Str.vi"("PF Channel"="PF Channel 25", "PF Card"="PF Card 25", "PF Chassis"="PF Chassis 25") -> ("PF Info"=w2810:string)
        n2140 = call "16CHDAQ - PF Info Num2Str.vi"("PF Channel"="PF Channel 26", "PF Card"="PF Card 26", "PF Chassis"="PF Chassis 26") -> ("PF Info"=w2809:string)
        n2141 = call "16CHDAQ - PF Info Num2Str.vi"("PF Channel"="PF Channel 27", "PF Card"="PF Card 27", "PF Chassis"="PF Chassis 27") -> ("PF Info"=w2808:string)
        n2142 = call "16CHDAQ - PF Info Num2Str.vi"("PF Channel"="PF Channel 28", "PF Card"="PF Card 28", "PF Chassis"="PF Chassis 28") -> ("PF Info"=w2807:string)
        n2143 = call "16CHDAQ - PF Info Num2Str.vi"("PF Channel"="PF Channel 29", "PF Card"="PF Card 29", "PF Chassis"="PF Chassis 29") -> ("PF Info"=w2806:string)
        n2144 = call "16CHDAQ - PF Info Num2Str.vi"("PF Channel"="PF Channel 30", "PF Card"="PF Card 30", "PF Chassis"="PF Chassis 30") -> ("PF Info"=w2805:string)
        n2145 = call "16CHDAQ - PF Info Num2Str.vi"("PF Channel"="PF Channel 31", "PF Card"="PF Card 31", "PF Chassis"="PF Chassis 31") -> ("PF Info"=w2804:string)
        n2146 = Bundle("Sensitivity 0"="Sensitivity 0", "Sensitivity 1"="Sensitivity 1", "Sensitivity 2"="Sensitivity 2", "Sensitivity 3"="Sensitivity 3", "Sensitivity 4"="Sensitivity 4", "Sensitivity 5"="Sensitivity 5", "Sensitivity 6"="Sensitivity 6", "Sensitivity 7"="Sensitivity 7", "Sensitivity 8"="Sensitivity 8", "Sensitivity 9"="Sensitivity 9", "Sensitivity 10"="Sensitivity 10", "Sensitivity 11"="Sensitivity 11", "Sensitivity 12"="Sensitivity 12", "Sensitivity 13"="Sensitivity 13", "Sensitivity 14"="Sensitivity 14", "Sensitivity 15"="Sensitivity 15", "Sensitivity 16"="Sensitivity 16", "Sensitivity 17"="Sensitivity 17", "Sensitivity 18"="Sensitivity 18", "Sensitivity 19"="Sensitivity 19", "Sensitivity 20"="Sensitivity 20", "Sensitivity 21"="Sensitivity 21", "Sensitivity 22"="Sensitivity 22", "Sensitivity 23"="Sensitivity 23", "Sensitivity 24"="Sensitivity 24", "Sensitivity 25"="Sensitivity 25", "Sensitivity 26"="Sensitivity 26", "Sensitivity 27"="Sensitivity 27", "Sensitivity 28"="Sensitivity 28", "Sensitivity 29"="Sensitivity 29", "Sensitivity 30"="Sensitivity 30", "Sensitivity 31"="Sensitivity 31") -> (w2985:T50)  [unwired: 1 in]
        n2147 = Bundle("PF Info"=w3152, "PF Info"=w3156, "PF Info"=w3162, "PF Info"=w3166, "PF Info"=w3170, "PF Info"=w3174, "PF Info"=w3178, "PF Info"=w3182, "PF Info"=w3186, "PF Info"=w3215, "PF Info"=w3216, "PF Info"=w3217, "PF Info"=w3218, "PF Info"=w3219, "PF Info"=w3220, "PF Info"=w3221, "PF Info"=w2819, "PF Info"=w2818, "PF Info"=w2817, "PF Info"=w2816, "PF Info"=w2815, "PF Info"=w2814, "PF Info"=w2813, "PF Info"=w2812, "PF Info"=w2811, "PF Info"=w2810, "PF Info"=w2809, "PF Info"=w2808, "PF Info"=w2807, "PF Info"=w2806, "PF Info"=w2805, "PF Info"=w2804) -> (w2979:T63)  [unwired: 1 in]
        n2148 = Bundle("PF Condition 0"="PF Condition 0", "PF Condition 1"="PF Condition 1", "PF Condition 2"="PF Condition 2", "PF Condition 3"="PF Condition 3", "PF Condition 4"="PF Condition 4", "PF Condition 5"="PF Condition 5", "PF Condition 6"="PF Condition 6", "PF Condition 7"="PF Condition 7", "PF Condition 8"="PF Condition 8", "PF Condition 9"="PF Condition 9", "PF Condition 10"="PF Condition 10", "PF Condition 11"="PF Condition 11", "PF Condition 12"="PF Condition 12", "PF Condition 13"="PF Condition 13", "PF Condition 14"="PF Condition 14", "PF Condition 15"="PF Condition 15", "PF Condition 16"="PF Condition 16", "PF Condition 17"="PF Condition 17", "PF Condition 18"="PF Condition 18", "PF Condition 19"="PF Condition 19", "PF Condition 20"="PF Condition 20", "PF Condition 21"="PF Condition 21", "PF Condition 22"="PF Condition 22", "PF Condition 23"="PF Condition 23", "PF Condition 24"="PF Condition 24", "PF Condition 25"="PF Condition 25", "PF Condition 26"="PF Condition 26", "PF Condition 27"="PF Condition 27", "PF Condition 28"="PF Condition 28", "PF Condition 29"="PF Condition 29", "PF Condition 30"="PF Condition 30", "PF Condition 31"="PF Condition 31") -> (w2980:T54)  [unwired: 1 in]
        n2149 = Bundle("Physical Channels Ch 0"="Physical Channels Ch 0", "Physical Channel Ch 1"="Physical Channel Ch 1", "Physical Channel Ch 2"="Physical Channel Ch 2", "Physical Channels Ch 3"="Physical Channels Ch 3", "Physical Channel Ch 4"="Physical Channel Ch 4", "Physical Channel Ch 5"="Physical Channel Ch 5", "Physical Channels Ch 6"="Physical Channels Ch 6", "Physical Channel Ch 7"="Physical Channel Ch 7", "Physical Channel Ch 8"="Physical Channel Ch 8", "Physical Channel Ch 9"="Physical Channel Ch 9", "Physical Channel Ch 10"="Physical Channel Ch 10", "Physical Channel Ch 11"="Physical Channel Ch 11", "Physical Channel Ch 12"="Physical Channel Ch 12", "Physical Channel Ch 13"="Physical Channel Ch 13", "Physical Channel Ch 14"="Physical Channel Ch 14", "Physical Channel Ch 15"="Physical Channel Ch 15", "Physical Channel Ch 16"="Physical Channel Ch 16", "Physical Channel Ch 17"="Physical Channel Ch 17", "Physical Channel Ch 18"="Physical Channel Ch 18", "Physical Channel Ch 19"="Physical Channel Ch 19", "Physical Channel Ch 20"="Physical Channel Ch 20", "Physical Channel Ch 21"="Physical Channel Ch 21", "Physical Channel Ch 22"="Physical Channel Ch 22", "Physical Channel Ch 23"="Physical Channel Ch 23", "Physical Channel Ch 24"="Physical Channel Ch 24", "Physical Channel Ch 25"="Physical Channel Ch 25", "Physical Channel Ch 26"="Physical Channel Ch 26", "Physical Channel Ch 27"="Physical Channel Ch 27", "Physical Channel Ch 28"="Physical Channel Ch 28", "Physical Channel Ch 29"="Physical Channel Ch 29", "Physical Channel Ch 30"="Physical Channel Ch 30", "Physical Channel Ch 31"="Physical Channel Ch 31") -> (w2988:T64)  [unwired: 1 in]
        n2150 = property on="Striker Velocity (m/s)" class="DigNum (strict)"() -> ("Value"=w3040:dbl)  [unwired: 2 in, 2 out]
        n2151 = property on="Trigger (Yes if on)" class="Bool (strict)"() -> ("Value"=w2768:bool)  [unwired: 2 in, 2 out]
        n2152 = case shown="False" w2768 {
          tunnel: [w3268 w3269] -> w3039
          frame False {
            n2153 = property on="Sample Rate (Sa/sec)" class="DigNum (strict)"() -> ("Value"=w3268:dbl)  [unwired: 2 in, 2 out]
          }
          frame True {
            n2154 = property on="Sample Rate (Sa/sec)" class="DigNum (strict)"() -> ("Value"=w3269:dbl)  [unwired: 2 in, 2 out]
          }
        }
        n2155 = Bundle("Programmer Info"="Programmer Info", "Value"=w3040, "Value"=w3039) -> (w2803:T5)  [unwired: 1 in]
        "Save Info" <- w2803
        n2156 = Bundle(w2989, w2990, w2988, w2987, w2986, w2985, w2984, w2983, w2982, w2981, w2980, w2979) -> (w2769:T2)  [unwired: 1 in]
        "output cluster 3" <- w2769
        n2157 = property on="output cluster" class="Clust (strict)"("Value"=w2769) -> ()  [unwired: 2 in, 2 out]
        n2158 = Bundle(w2769, w2803) -> ()  [unwired: 1 in, 1 out]
      }
    }
    n2159 = Equal?(x=w6, y=32CHDAQ_-_Cases."End" ("Program State")) -> (x = y?=w10:bool)
  }
